vi "Get Ctrl Info.vi"(8 "error in (no error)":errorcluster, 9 "GObj Refnum":refnum<vi>, 10 "VI-Ref":refnum<vi>, 11 "Ctrl Reference's in":refnum<class "Ctrl Reference's.lvclass">) -> (0 "error out":errorcluster, 1 "Has Label?":bool, 2 "Label":string, 3 "Ctrl Reference's out":refnum<class "Ctrl Reference's.lvclass">)   [LabVIEW 2025, in "Ctrl Reference's.lvclass"]
uses:
  Ctrl Reference's.lvclass
  Ctrl Reference's.lvclass/Ctrl Reference's.ctl
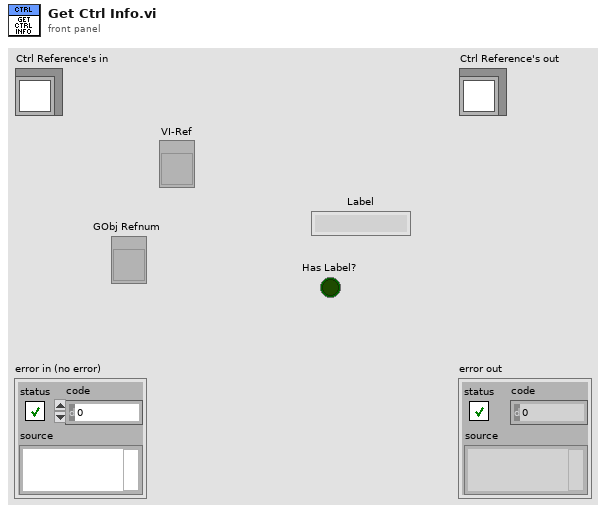
[diagram p1: front panel]
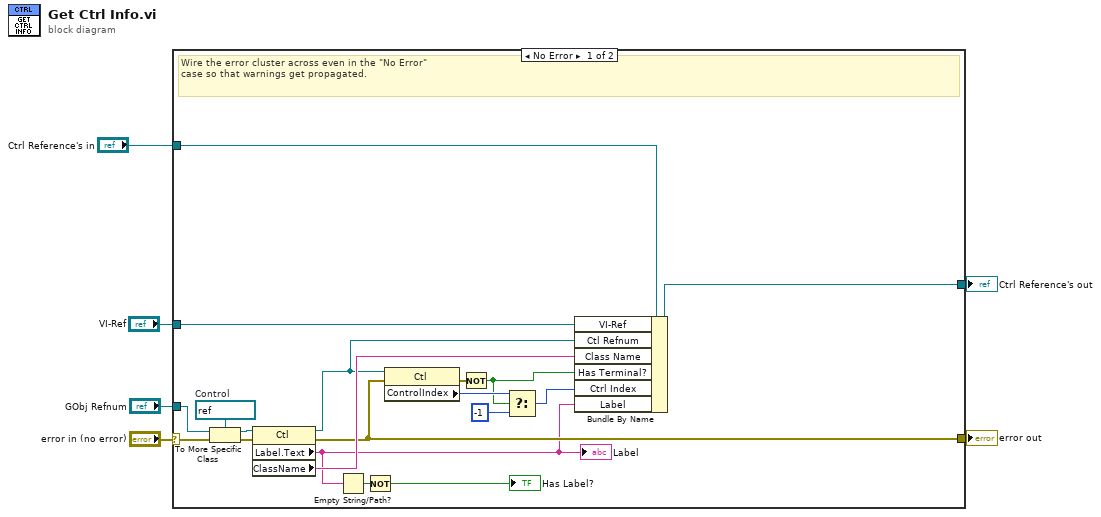
[diagram p0: block diagram]
diagram:
  n1 = case shown="No Error" "error in (no error)" {
    selector: "error in (no error)" -> [w16 w27]
    tunnel: [w11 w27] -> w5
    tunnel: [w24 w26] -> w3
    tunnel: "Ctrl Reference's in" -> [w25 w26]
    tunnel: "GObj Refnum" -> [w15 _]
    tunnel: "VI-Ref" -> [w9 _]
    frame No Error {
      w23 = refnum<vi> refnum  # Control
      # "Wire the error cluster across even in the \"No Error\"\ncase so that warnings get propagated."
      n2 = To More Specific Class(target class=w23, reference=w15, error in=w16) -> (specific class reference=w22:refnum<vi>, error out=w21:errorcluster)
      n3 = property class="Ctl"(reference=w22, error in=w21) -> (reference out=w7:refnum<vi>, error out=w11:errorcluster, "Label.Text"=w8:string, "ClassName"=w14:string)
      "Label" <- w8
      n4 = Empty String/Path?(string/path=w8) -> (empty?=w20:bool)
      n5 = Not(x=w20) -> (.not. x?=→"Has Label?":bool)
      n6 = property class="Ctl"(reference=w7, error in=w11) -> (error out=w19:errorcluster, "ControlIndex"=w18:i32)  [unwired: 1 out]
      n7 = Not(x=w19) -> (.not. x?=w13:bool)
      n8 = Select(t=w18, s=w13, f=-1) -> (s? t:f=w12:i32)
      n9 = Bundle By Name(cluster=w25, "VI-Ref"=w9, "Ctl Refnum"=w7, "Class Name"=w14, "Has Terminal?"=w13, "Ctrl Index"=w12, "Label"=w8) -> (w24:refnum<class "Ctrl Reference's.lvclass">)
    }
    frame Error {
    }
  }
  "error out" <- w5
  "Ctrl Reference's out" <- w3
